vi "Write Address.lvclass.vi"(8 "error in (no error)":errorcluster, 10 "Address.lvclass":refnum<class "Address.lvclass">, 11 "Speed Mode in":refnum<class "Speed Mode.lvclass">) -> (0 "error out":errorcluster, 3 "Speed Mode out":refnum<class "Speed Mode.lvclass">)   [LabVIEW 2020, in "Speed Mode.lvclass"]
uses:
  Speed Mode.lvclass
  Address/Address.lvclass
  Speed Mode.lvclass/Speed Mode.ctl
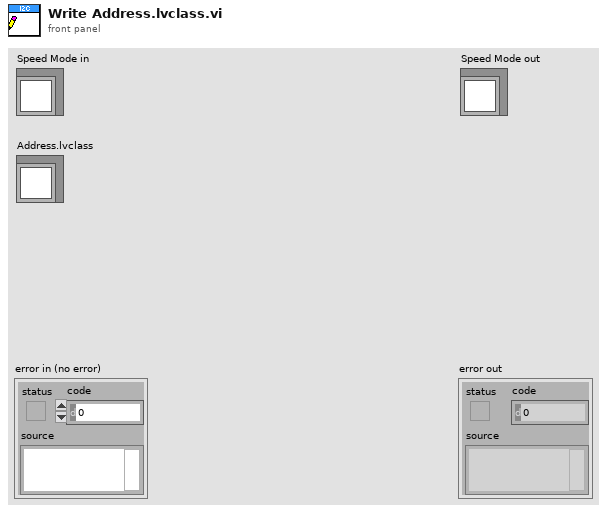
[diagram p1: front panel]
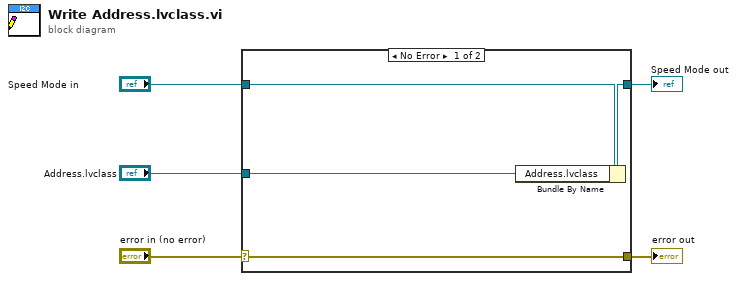
[diagram p0: block diagram]
diagram:
  n1 = case shown="No Error" "error in (no error)" {
    selector: "error in (no error)" -> [w9 w10]
    tunnel: [w9 w10] -> w4
    tunnel: [w7 w11] -> w2
    tunnel: "Speed Mode in" -> [w8 w11]
    tunnel: "Address.lvclass" -> [w6 _]
    frame No Error {
      n2 = Bundle By Name(cluster=w8, "Address.lvclass"=w6) -> (w7:refnum<class "Speed Mode.lvclass">)
    }
    frame Error {
    }
  }
  "error out" <- w4
  "Speed Mode out" <- w2
